vi "onDependencyConfigChanged.vi"(4 "Source GUID":string, 6 "keys changed":string[](array[string]), 7 "Propagate to caller? (T)":bool=TRUE, 8 "error in":errorcluster, 9 "Dependency":refnum<class "SMO.lvclass">, 11 "SMO.Configurable in":refnum<class "SMO.Configurable.lvclass">) -> (0 "error out":errorcluster, 3 "SMO.Configurable out":refnum<class "SMO.Configurable.lvclass">)   [LabVIEW 2013, in "SMO.Configurable.lvclass"]
uses:
  SMO.Configurable.lvclass
  src/SMO/SMO.lvclass
  SMO.Configurable.lvclass/SMO.Configurable.ctl
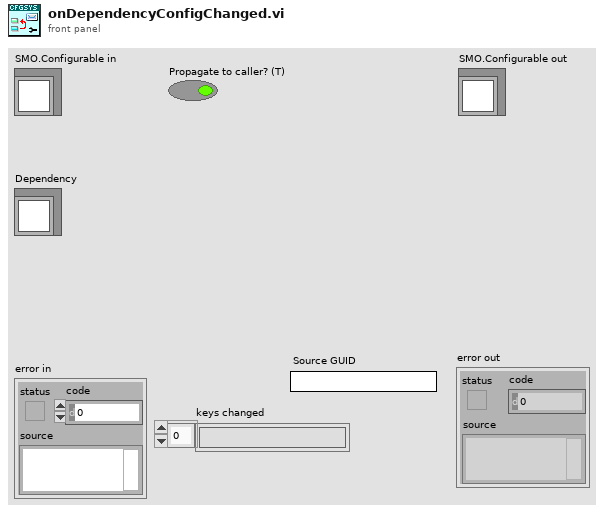
[diagram p1: front panel]
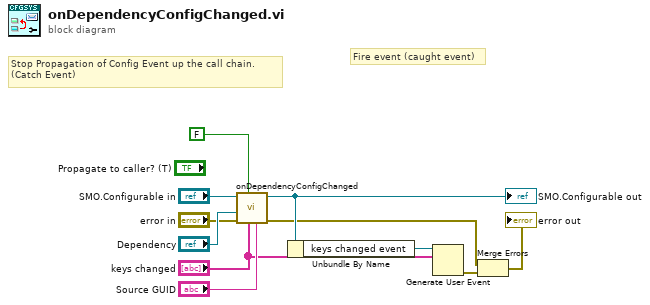
[diagram p0: block diagram]
diagram:
  # "Fire event (caught event)"
  # "Stop Propagation of Config Event up the call chain.\n(Catch Event)"
  n1 = call-parent "onDependencyConfigChanged.vi"("Source GUID"="Source GUID", "keys changed"="keys changed", "Propagate to caller? (T)"=FALSE, "error in"="error in", "Dependency"="Dependency", "SMO in"="SMO.Configurable in") -> ("error out"=w3:errorcluster, "SMO out"=w7:refnum<class "SMO.Configurable.lvclass">)  [unwired: 4 in]
  "SMO.Configurable out" <- w7
  n2 = Unbundle By Name(w7) -> ("keys changed event"=w6:refnum<user-event>)
  n3 = Generate User Event(user event=w6, event data cluster="keys changed") -> (error out=w4:errorcluster)  [unwired: 2 in, 1 out]
  n4 = Merge Errors(w3, w4) -> (→"error out":errorcluster)
